vi "Update Message Count.vi"(8 "error in (no error)":errorcluster, 10 "Value":i32, 11 "DigNum in":refnum<vi>) -> (0 "error out":errorcluster)   [LabVIEW 2025, in "I2C Bus Monitor.lvclass"]
uses:
  I2C Bus Monitor.lvclass
  I2C Bus Monitor.lvclass/I2C Bus Monitor.ctl
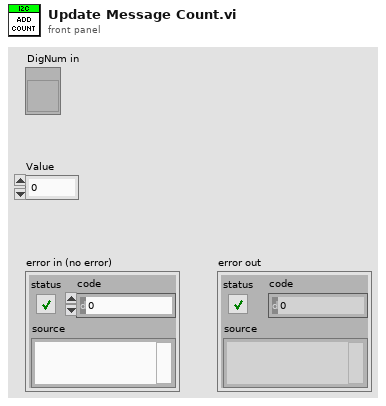
[diagram p1: front panel]
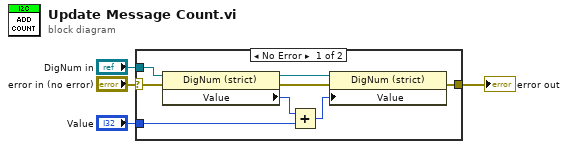
[diagram p0: block diagram]
diagram:
  n1 = case shown="No Error" "error in (no error)" {
    selector: "error in (no error)" -> [w11 w13]
    tunnel: "DigNum in" -> [w12 _]
    tunnel: [w10 w13] -> w3
    tunnel: "Value" -> [w5 _]
    frame No Error {
      n2 = property on="Property Node" class="DigNum (strict)"(reference=w12, error in=w11) -> (reference out=w7:refnum<vi>, error out=w6:errorcluster, "Value"=w8:i32)
      n3 = Add(x=w8, y=w5) -> (x+y=w9:i32)
      n4 = property on="Property Node" class="DigNum (strict)"(reference=w7, error in=w6, "Value"=w9) -> (error out=w10:errorcluster)  [unwired: 1 out]
    }
    frame Error {
    }
  }
  "error out" <- w3
